vi "XXX Result to XML.vi"(8 "error in (no error)":errorcluster, 9 "Test Result":T1={"#attributes"={"Version"="MTE_1.0.0"}, "Facility"={"Name"="", "Location"=""}, "Station"={"Name"="", "PN"="", "SN"="", "Rev"="", "PC Name"="", "Location"="", "HW_Config"={"HW_Item"=[]}, "SW_Config"={"SW_Item"=[]}}, "Test Run"={"Operator"="", "Start Time"=timestamp(0 s since 1904-01-01), "Duration(s)"=0.0, "Mode"="", "Comment"="", "ProcessStep"=""}, "Test Sequence"={"Name"="", "Config"={"Config_Item"=[]}}, "UUTs"={"UUT"=[]}} {"UUTs"."UUT"."Attributes"."Attribute"."Status" items=["LOG", "PASS", "FAIL", "ERROR"]; "UUTs"."UUT"."Measurements"."Measurement"."Status" items=["LOG", "PASS", "FAIL", "ERROR"]}, 11 "Path":path) -> (0 "error out":errorcluster)   [LabVIEW 2018]
uses:
  TestResult.Facility.ctl
  TestResult.SW Item.ctl
  TestResult.HW Item.ctl
  TestResult.Station Info.ctl
  TestResult.Symptom.State.ctl
  TestResult.Test Run Info.ctl
  Result.Numeric.ctl
  TestResult.UUT Result.ctl
  TestResult.Symptom.ctl
  TestResult.Test Info.ctl
  TestResult.FullResultData.ctl
  Result.Attribute.ctl
  Result.Measurement and Attribute Item Status.ctl
  Result.Limit Type.ctl
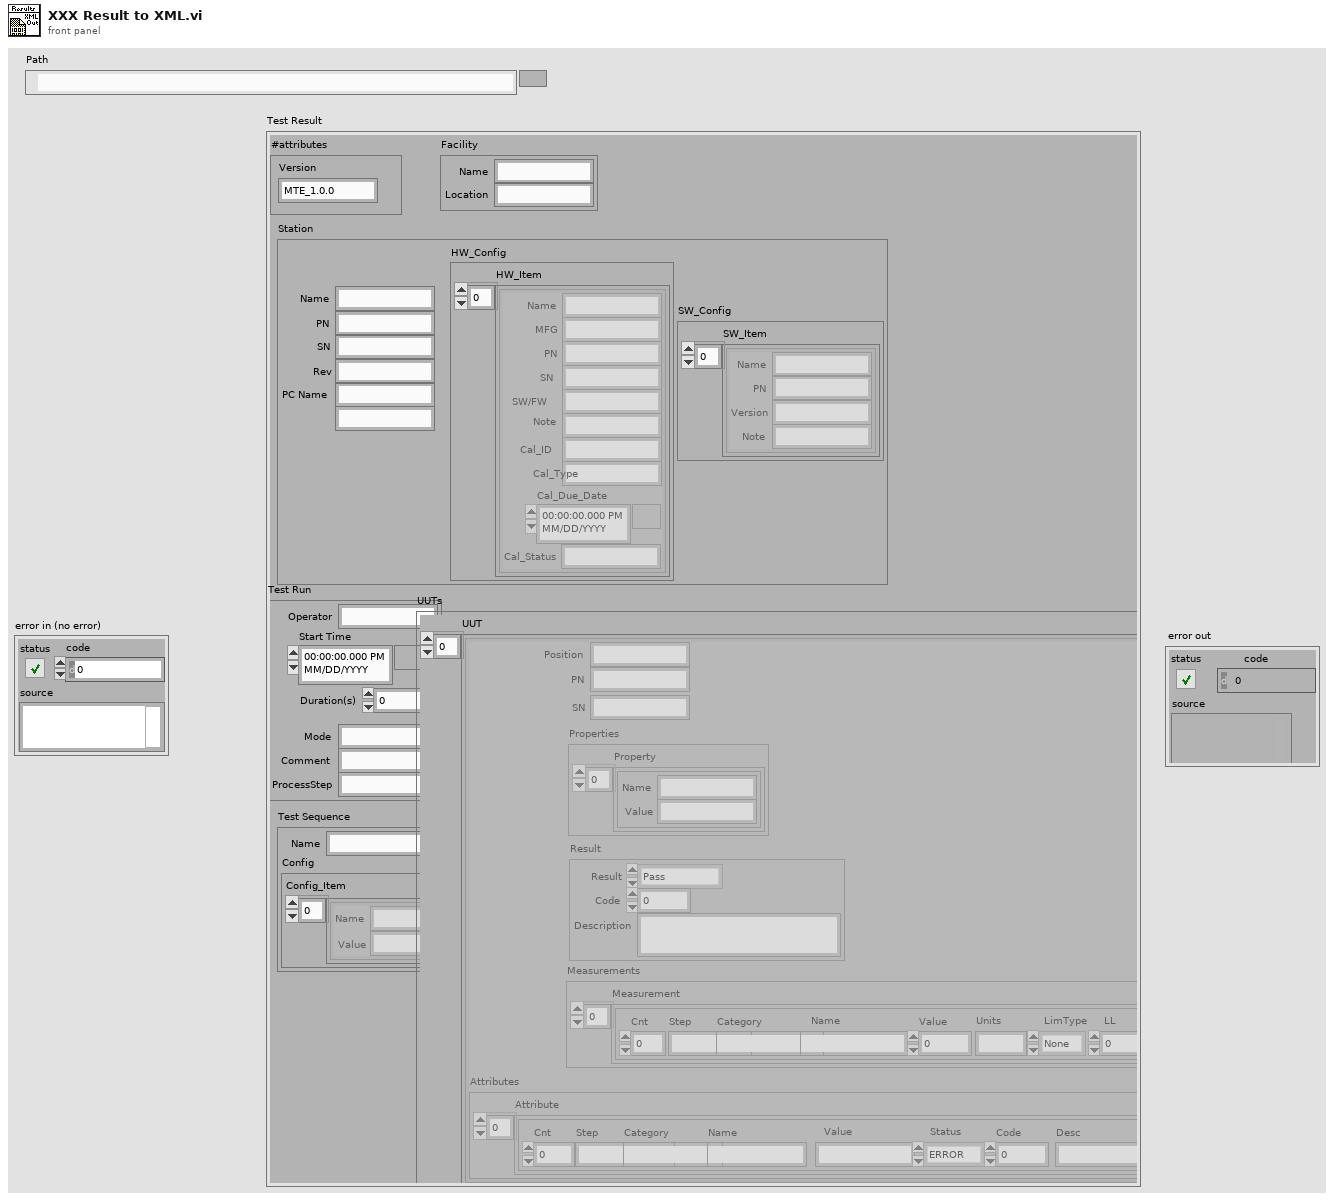
[diagram p1: front panel]
types:
  T1 = typedef "TestResult.FullResultData.ctl" = cluster{"#attributes":cluster{"Version":string}, "Facility":T2, "Station":T3, "Test Run":T6, "Test Sequence":T7, "UUTs":cluster{"UUT":T8[]}}
  T2 = typedef "TestResult.Facility.ctl" = cluster{"Name":string, "Location":string}
  T3 = typedef "TestResult.Station Info.ctl" = cluster{"Name":string, "PN":string, "SN":string, "Rev":string, "PC Name":string, "Location":string, "HW_Config":cluster{"HW_Item":T4[]}, "SW_Config":cluster{"SW_Item":T5[]}}
  T4 = typedef "TestResult.HW Item.ctl" = cluster{"Name":string, "MFG":string, "PN":string, "SN":string, "SW/FW":string, "Note":string, "Cal_ID":string, "Cal_Type":string, "Cal_Due_Date":timestamp, "Cal_Status":string}
  T5 = typedef "TestResult.SW Item.ctl" = cluster{"Name":string, "PN":string, "Version":string, "Note":string}
  T6 = typedef "TestResult.Test Run Info.ctl" = cluster{"Operator":string, "Start Time":timestamp, "Duration(s)":dbl, "Mode":string, "Comment":string, "ProcessStep":string}
  T7 = typedef "TestResult.Test Info.ctl" = cluster{"Name":string, "Config":cluster{"Config_Item":cluster{"Name":string, "Value":string}[]}}
  T8 = typedef "TestResult.UUT Info.ctl" = cluster{"Position":string, "PN":string, "SN":string, "Properties":cluster{"Property":cluster{"Name":string, "Value":string}[]}, "Result":T9, "Measurements":cluster{"Measurement":T11[]}, "Attributes":cluster{"Attribute":T14[]}}
  T9 = typedef "TestResult.Symptom.ctl" = cluster{"Result":T10, "Code":i32, "Description":string}
  T10 = typedef "TestResult.Symptom.State.ctl" = enum16{"Pass", "Fail", "Error", "Aborted", "Completed", "Logged"}
  T11 = typedef "Result.Numeric.ctl" = cluster{"Cnt":i32, "Step":string, "Category":string, "Name":string, "Value":dbl, "Units":string, "LimType":T12, "LL":dbl, "UL":dbl, "Status":T13, "Code":i32, "Desc":string, "Time":timestamp}
  T12 = typedef "Result.Limit Type.ctl" = enum16{"None", "EQ", "NE", "GT", "LT", "GE", "LE", "GTLT", "GELE", "GELT", "GTLE", "LTGT", "LEGE", "LEGT", "LTGE"}
  T13 = typedef "Result.Measurement and Attribute Item Status.ctl" = i32
  T14 = typedef "Result.Attribute.ctl" = cluster{"Cnt":i32, "Step":string, "Category":string, "Name":string, "Value":string, "Status":T13, "Code":i32, "Desc":string, "Time":timestamp}
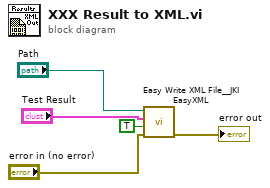
[diagram p0: block diagram]
diagram:
  n1 = call <vilib>:"Easy Write XML File__JKI EasyXML.vi"("error in (no error)"="error in (no error)", "Overwrite File? (false)"=TRUE, "LabVIEW Data"="Test Result", "XML File Path"="Path") -> ("error out"=→"error out":errorcluster)  [unwired: 6 in, 1 out]
